vi "Ex12 Shape Detection.vi"() -> ()   [LabVIEW 2020]
panel:
  out "Coordinate System Out (Set Coordinate System 2)":T1 {"Measurement System"."Axis Reference" items=["Direct", "Indirect"]; "Measurement System"."Angle (deg)" format="%.2f"; "Measurement System"."Origin"."Y" format="%.2f"; "Measurement System"."Origin"."X" format="%.2f"; "Reference System"."Axis Reference" items=["Direct", "Indirect"]; "Reference System"."Angle (deg)" format="%.2f"; "Reference System"."Origin"."Y" format="%.2f"; "Reference System"."Origin"."X" format="%.2f"}
  out "Coordinate System Out (Set Coordinate System 1)":T1 {"Measurement System"."Axis Reference" items=["Direct", "Indirect"]; "Measurement System"."Angle (deg)" format="%.2f"; "Measurement System"."Origin"."Y" format="%.2f"; "Measurement System"."Origin"."X" format="%.2f"; "Reference System"."Axis Reference" items=["Direct", "Indirect"]; "Reference System"."Angle (deg)" format="%.2f"; "Reference System"."Origin"."Y" format="%.2f"; "Reference System"."Origin"."X" format="%.2f"}
  out "error out":errorcluster
  out "Processed Image":T2(plugin-control)
  out "Image":T2(plugin-control)
  in  "File Path":path
  # "EX.12 SHAPE DETECTION"
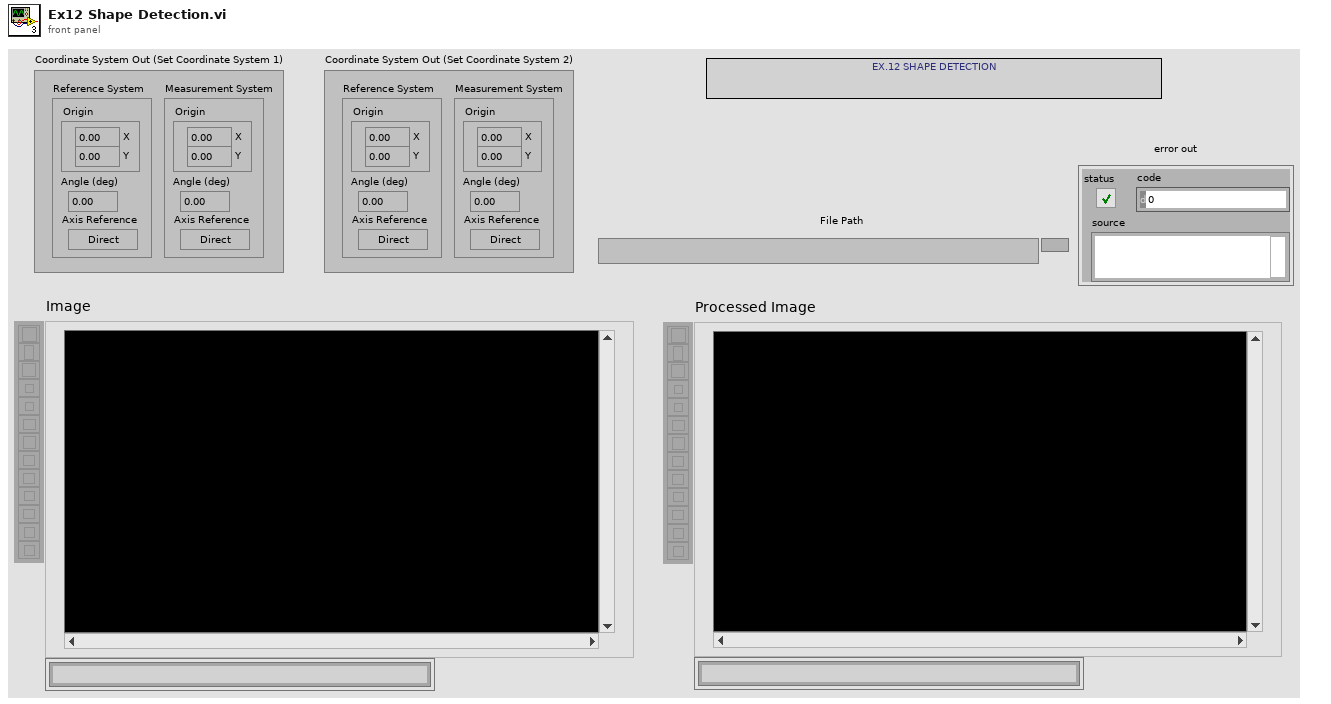
[diagram p1: front panel]
types:
  T1 = cluster{"Reference System":cluster{"Origin":cluster{"X":sgl, "Y":sgl}, "Angle (deg)":sgl, "Axis Reference":u32}, "Measurement System":cluster{"Origin":cluster{"X":sgl, "Y":sgl}, "Angle (deg)":sgl, "Axis Reference":u32}}
  T2 = typedef "IMAQ Image.ctl" = refnum<image>
  T3 = typedef "Image Type" = u32
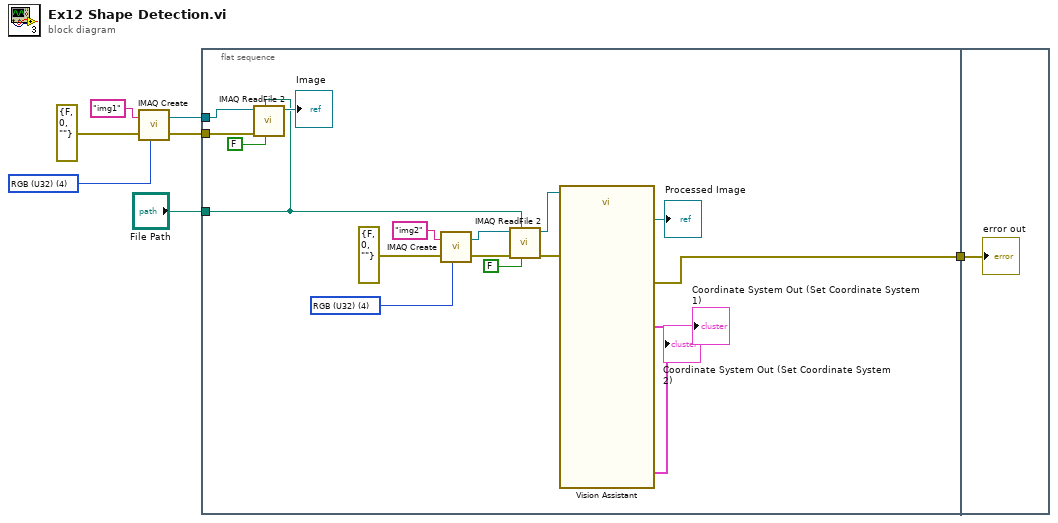
[diagram p0: block diagram]
diagram:
  w1 = T3 4 items=["Grayscale (U8)", "Grayscale (I16)", "Grayscale (SGL)", "Complex (CSG)", "RGB (U32)", "HSL (U32)", "RGB (U64)", "Grayscale (U16)"] ("Image Type")
  n1 = call "IMAQ Create"("Image Name"="img1", "Image Type"=w1, "error in (no error)"=errorcluster {"status"=FALSE, "code"=0, "source"=""}) -> ("New Image"=w2:T2, "error out"=w3:errorcluster)  [unwired: 2 in]
  n2 = flat-sequence {
    tunnel: "File Path" -> [w14]
    tunnel: w3 -> [w23]
    tunnel: w2 -> [w22]
    tunnel: [w10] -> w7
    tunnel: w7 -> [w25]
    frame #0 {
      w18 = T3 4 items=["Grayscale (U8)", "Grayscale (I16)", "Grayscale (SGL)", "Complex (CSG)", "RGB (U32)", "HSL (U32)", "RGB (U64)", "Grayscale (U16)"] ("Image Type")
      n3 = call "IMAQ ReadFile 2"("Use File Path Image Type"=FALSE, "File Path"=w14, "error in (no error)"=w23, "Image"=w22) -> ("Image Out"=→"Image":T2)  [unwired: 3 in, 4 out]
      n4 = call "IMAQ Create"("Image Name"="img2", "Image Type"=w18, "error in (no error)"=errorcluster {"status"=FALSE, "code"=0, "source"=""}) -> ("New Image"=w17:T2, "error out"=w16:errorcluster)  [unwired: 2 in]
      n5 = call "IMAQ ReadFile 2"("Use File Path Image Type"=FALSE, "File Path"=w14, "error in (no error)"=w16, "Image"=w17) -> ("error out"=w12:errorcluster, "Image Out"=w13:T2)  [unwired: 3 in, 3 out]
      n6 = call "Vision Assistant"("Image In"=w13, "error in"=w12) -> ("Image Out"=→"Processed Image":T2, "Coordinate System Out (Set Coordinate System 1)"=→"Coordinate System Out (Set Coordinate System 1)":T1, "Coordinate System Out (Set Coordinate System 2)"=→"Coordinate System Out (Set Coordinate System 2)":T1, "error out"=w10:errorcluster)  [unwired: 22 in]
    }
    frame #1 {
      "error out" <- w25
    }
  }
